vi "progra 13.vi"() -> ()   [LabVIEW 2011]
panel:
  in  "stop":bool
  out "Foco":bool
  in  "On/Off":bool
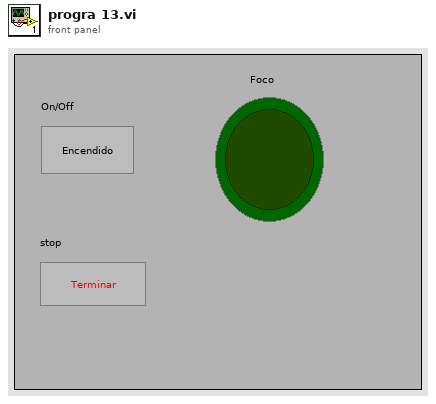
[diagram p1: front panel]
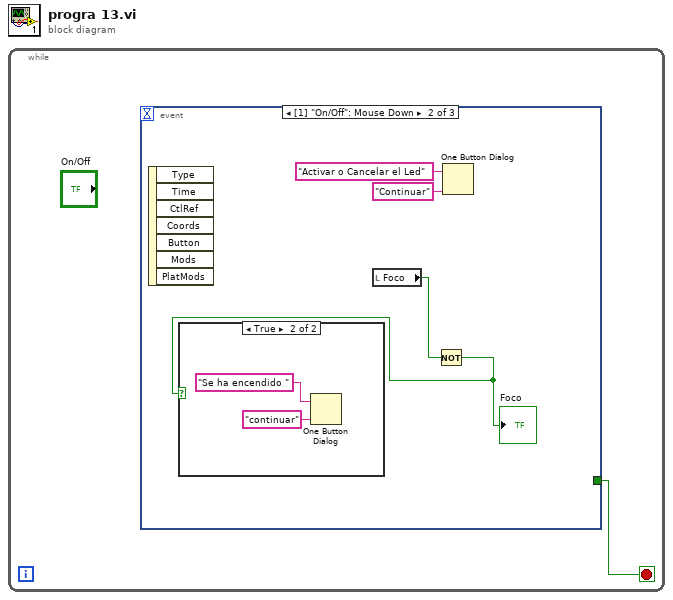
[diagram p0: block diagram]
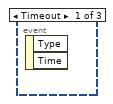
[diagram p2: hidden frame]
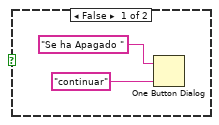
[diagram p3: hidden frame]
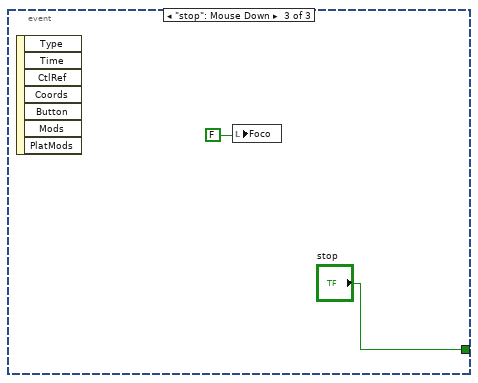
[diagram p4: hidden frame]
diagram:
  n1 = while {
    stop <- w1 stop-if-true
    n2 = event shown="[1] \"On/Off\": Mouse Down" {
      selector: _ -> [_ _ _]
      dyn-events: _ -> [_ _ _]
      timeout: _ -> [_ _ _]
      tunnel: [_ _ "stop"] -> w1
      event Timeout {
        n3 = event-data() -> ()  [unwired: 1 in, 2 out]
      }
      event "On/Off": Mouse Down {
        n4 = event-data() -> ()  [unwired: 1 in, 7 out]
        n5 = local read "Foco"() -> (w3:bool)
        n6 = Not(x=w3) -> (.not. x?=w2:bool)
        "Foco" <- w2
        n7 = case shown="True" w2 {
          frame False {
            n8 = One Button Dialog(message="Se ha Apagado ", button name ("OK")="continuar") -> ()  [unwired: 1 out]
          }
          frame True {
            n9 = One Button Dialog(message="Se ha encendido ", button name ("OK")="continuar") -> ()  [unwired: 1 out]
          }
        }
        n10 = One Button Dialog(message="Activar o Cancelar el Led", button name ("OK")="Continuar") -> ()  [unwired: 1 out]
      }
      event "stop": Mouse Down {
        n11 = event-data() -> ()  [unwired: 1 in, 7 out]
        n12 = local write "Foco"(FALSE) -> ()
      }
    }
  }
